vi "DMD_Sequence_Alloc_.vi"() -> ()   [LabVIEW 2020]
uses:
  <vilib>/Utility/error.llb/Error Cluster From Error Code.vi
  <userlib>/alp4395/alp4395.dll
panel:
  in  "TriggerPulseWidth":i32
  out "PicNum":i32
  in  "SequenceIdPtr Input":u32
  out "SequenceIdPtr":u32
  in  "DeviceIdPtr in":u32
  in  "error in (no error)":errorcluster
  out "Frequency (Hz)":dbl=17241379.310344826
  in  "Picture Time (μs)":i32
  in  "Illuminate Time (μs)":i32
  in  "Number of Frames":i32
  out "DeviceIdPtr out":u32
  out "error out":errorcluster={"status"=TRUE, "code"=8569, "source"="DMD_Sequence_Alloc.vi<ERR>\nAn error occurred initialising the ALP system.  Error codes are  1003 (Not Available), 1003 (Not Available),."}
  out "SequenceId":u32
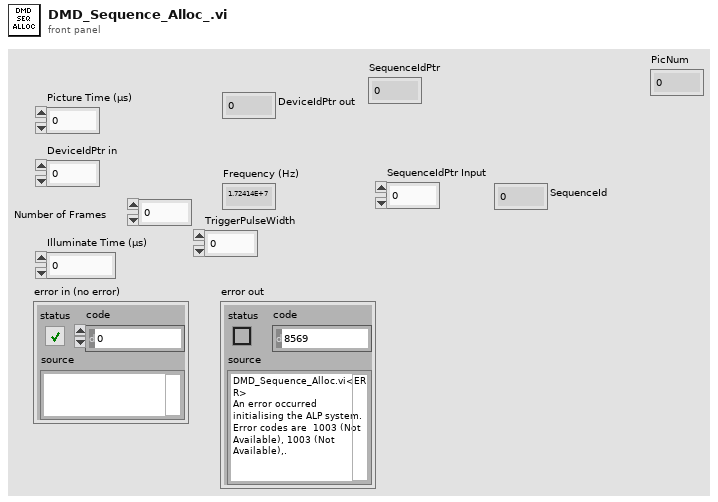
[diagram p1: front panel]
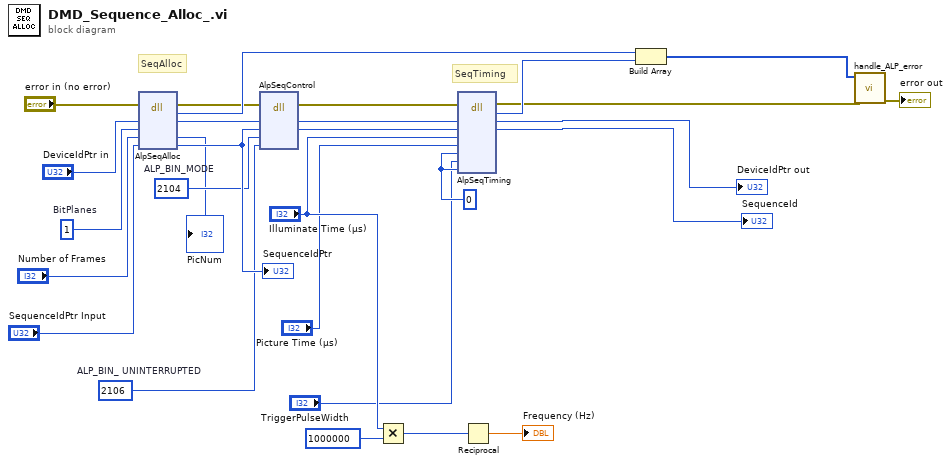
[diagram p0: block diagram]
diagram:
  w18 = 0 ("element")
  w10 = 2104  # ALP_BIN_MODE
  w9 = 2106  # ALP_BIN_ UNINTERRUPTED
  w16 = 1  # BitPlanes
  # "SeqTiming"
  # "SeqAlloc"
  n1 = dll-call lib="C:/Program Files (x86)/National Instruments/LabVIEW 2020/user.lib/alp4395/alp4395.dll" fn="AlpSeqAlloc"(error in="error in (no error)", "DeviceId"="DeviceIdPtr in", "BitPlanes"=w16, "PicNum"="Number of Frames", "SequenceIdPtr"="SequenceIdPtr Input") -> (error out=w13:errorcluster, "return type"=w24:i32, "DeviceId"=w12:u32, "PicNum"=→"PicNum":i32, "SequenceIdPtr"=w11:u32)  [unwired: 3 in, 1 out]
  "SequenceIdPtr" <- w11
  n2 = dll-call lib="C:/Program Files (x86)/National Instruments/LabVIEW 2020/user.lib/alp4395/alp4395.dll" fn="AlpSeqControl"(error in=w13, "DeviceId"=w12, "SequenceId"=w11, "ControlType"=w10, "ControlValue"=w9) -> (error out=w21:errorcluster, "DeviceId"=w22:u32, "SequenceId"=w23:u32)  [unwired: 5 in, 1 out]
  n3 = Multiply(x="Illuminate Time (μs)", y=1000000 ("element")) -> (x*y=w19:i32)
  n4 = dll-call lib="C:/Program Files (x86)/National Instruments/LabVIEW 2020/user.lib/alp4395/alp4395.dll" fn="AlpSeqTiming"(error in=w21, "DeviceId"=w22, "SequenceId"=w23, "IlluminateTime"="Illuminate Time (μs)", "PictureTime"="Picture Time (μs)", "TriggerDelay"=w18, "TriggerPulseWidth"="TriggerPulseWidth", "VdDelay"=w18) -> (error out=w5:errorcluster, "return type"=w25:i32, "DeviceId"=→"DeviceIdPtr out":u32, "SequenceId"=→"SequenceId":u32)  [unwired: 7 in, 1 out]
  n5 = Reciprocal(x=w19) -> (1/x=→"Frequency (Hz)":dbl)
  n6 = Build Array(w24, w25) -> (w27:i32[])
  n7 = call "handle_ALP_error.vi"("error in"=w5, "Return Codes"=w27) -> ("error out"=→"error out":errorcluster)  [unwired: 9 in]
